vi "CheckdRptFreq.vi"(8 "错误输入（无错误）":errorcluster, 11 "采样重复频率值":sgl) -> (0 "错误输出":errorcluster, 3 "返回值":i32)   [LabVIEW 2014]
uses:
  X86Dll/ZXUTConfigMgr.dll
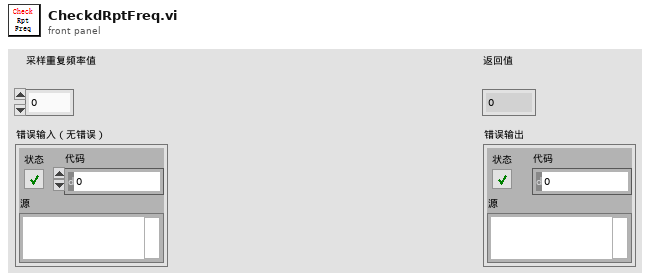
[diagram p1: front panel]
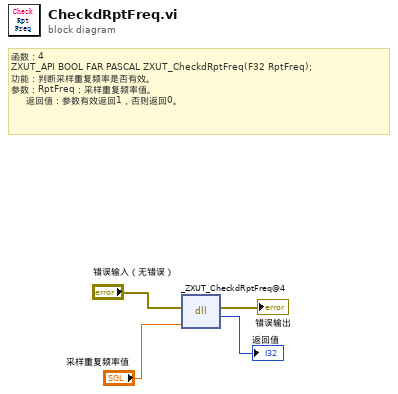
[diagram p0: block diagram]
diagram:
  # "函数：4\nZXUT_API BOOL\tFAR PASCAL ZXUT_CheckdRptFreq(F32 RptFreq);\n功能：判断采样重复频率是否有效。\n参数：RptFreq：采样重复频率值。\n\t    返回值：参数有效返回1，否则返回0。"
  n1 = dll-call lib="D:/Software/Utrasonic on-line monitoring/X86Dll/ZXUTConfigMgr.dll" fn="_ZXUT_CheckdRptFreq@4"(error in="错误输入（无错误）", "RptFreq"="采样重复频率值") -> (error out=→"错误输出":errorcluster, "返回值"=→"返回值":i32)  [unwired: 3 in, 1 out]
